vi "GV pixel sync.vi"() -> ()   [LabVIEW 2017]
panel:
  out "Pixel sync":bool
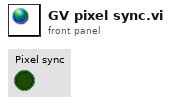
[diagram p1: front panel]
diagram:
